vi "Stop FGV.vi"(11 "Write?":bool) -> (3 "Stop?":bool)   [LabVIEW 2015]
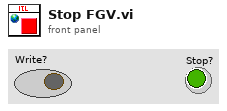
[diagram p1: front panel]
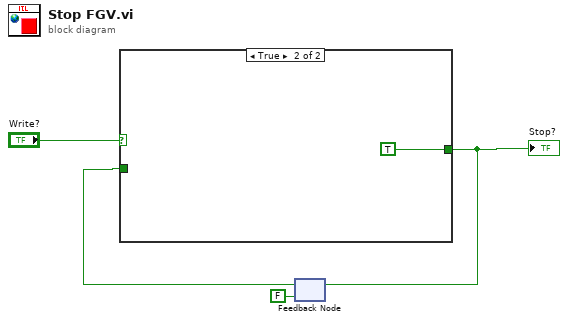
[diagram p0: block diagram]
diagram:
  n1 = feedback #1(FALSE) -> (w1:bool)
  n2 = case shown="True" "Write?" {
    tunnel: [w5 TRUE] -> w3
    tunnel: w1 -> [w5 _]
    frame False {
    }
    frame True {
    }
  }
  "Stop?" <- w3
  n3 = feedback-in #1(w3) -> ()
